vi "Set Color.vi"(8 "error in (no error)":errorcluster, 10 "Color":u16, 11 "Pixel in":refnum<class "Pixel.lvclass">) -> (0 "error out":errorcluster, 3 "Pixel out":refnum<class "Pixel.lvclass">)   [LabVIEW 2020, in "RPI.SenseHat.Display.lvlib" / "Pixel.lvclass"]
doc: "Sets the pixel color."
uses:
  Pixel.lvclass
  Pixel.lvclass/Pixel.ctl
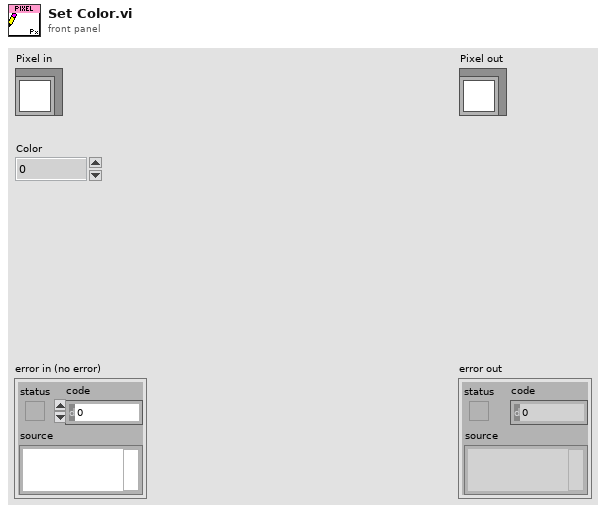
[diagram p1: front panel]
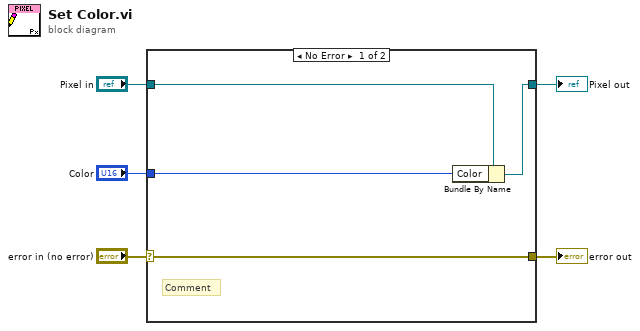
[diagram p0: block diagram]
diagram:
  n1 = case shown="No Error" "error in (no error)" {
    selector: "error in (no error)" -> [w9 w10]
    tunnel: [w9 w10] -> w4
    tunnel: [w7 w11] -> w2
    tunnel: "Pixel in" -> [w8 w11]
    tunnel: "Color" -> [w6 _]
    frame No Error {
      # "Comment"
      n2 = Bundle By Name(cluster=w8, "Color"=w6) -> (w7:refnum<class "Pixel.lvclass">)
    }
    frame Error {
    }
  }
  "error out" <- w4
  "Pixel out" <- w2
